vi "Basic Binding Test.vi"() -> (0 "error out":errorcluster)   [LabVIEW 2014, in "SQLite3LV Tests.lvlib"]
uses:
  SQLite3LV Tests.lvlib
  SQLite3LV/SQLite3 Class/struct_table_info.ctl
  SQLite3LV/Cursor Class/property binding/bind text.vi
  SQLite3LV/SQLite3 Class/sqlite3.lvclass
  SQLite3LV/Cursor Class/cursor.lvclass
  SQLite3LV/SQLite3LV.lvlib
panel:
  out "table info.":T1[](array[typedef])
  out "result":string[][](array[string])
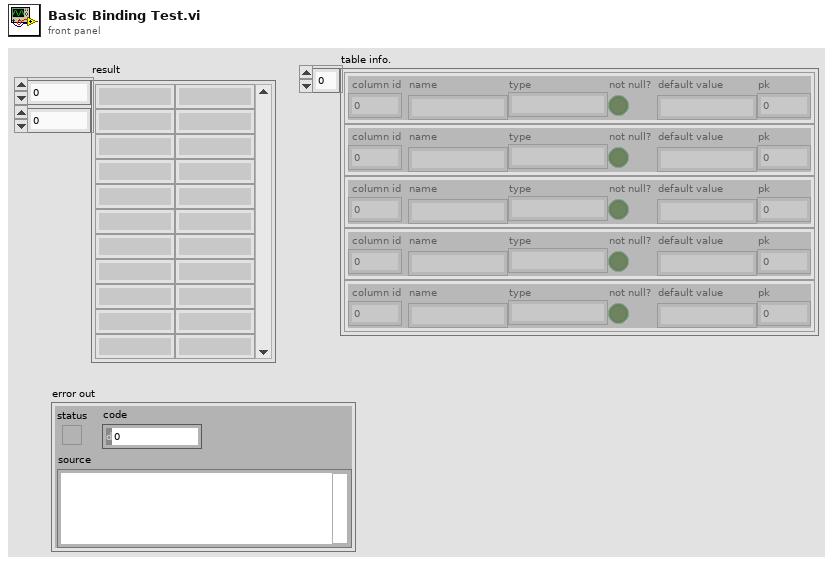
[diagram p1: front panel]
types:
  T1 = typedef "SQLite3LV.lvlib/struct_table_info.ctl" = cluster{" column id":i32, "name":string, "type":string, "not null?":bool, "default value":string, "pk":i32}
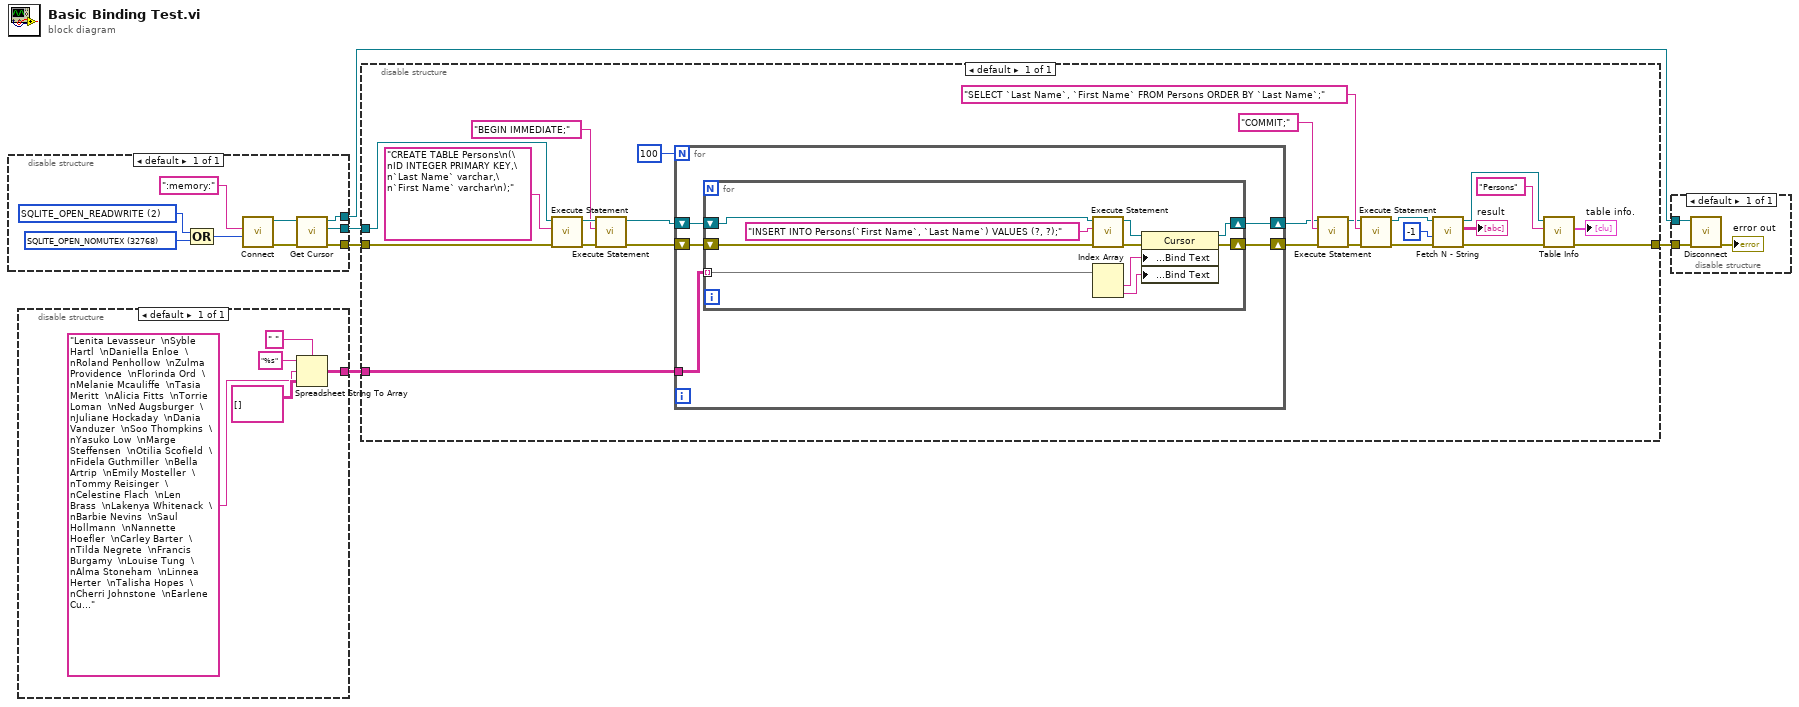
[diagram p0: block diagram]
diagram:
  n1 = disable-structure shown="default" {
    disable-tunnel: [w9] -> w5
    disable-tunnel: [w8] -> w4
    disable-tunnel: [w7] -> w3
    frame Enabled {
      w13 = u32 32768 items=["SQLITE_OPEN_READONLY"=1, "SQLITE_OPEN_READWRITE"=2, "SQLITE_OPEN_CREATE"=4, "SQLITE_OPEN_DELETEONCLOSE"=8, "SQLITE_OPEN_EXCLUSIVE"=16, "SQLITE_OPEN_AUTOPROXY"=32, "SQLITE_OPEN_URI"=64, "SQLITE_OPEN_MEMORY"=128, "SQLITE_OPEN_MAIN_DB"=256, "SQLITE_OPEN_TEMP_DB"=512, "SQLITE_OPEN_TRANSIENT_DB"=1024, "SQLITE_OPEN_MAIN_JOURNAL"=2048, "SQLITE_OPEN_TEMP_JOURNAL"=4096, "SQLITE_OPEN_SUBJOURNAL"=8192, "SQLITE_OPEN_MASTER_JOURNAL"=16384, "SQLITE_OPEN_NOMUTEX"=32768, "SQLITE_OPEN_FULLMUTEX"=65536, "SQLITE_OPEN_SHAREDCACHE"=131072, "SQLITE_OPEN_PRIVATECACHE"=262144, "SQLITE_OPEN_WAL"=524288] ("SQLITE3 Open Flag")
      w14 = u32 2 items=["SQLITE_OPEN_READONLY"=1, "SQLITE_OPEN_READWRITE"=2, "SQLITE_OPEN_CREATE"=4, "SQLITE_OPEN_DELETEONCLOSE"=8, "SQLITE_OPEN_EXCLUSIVE"=16, "SQLITE_OPEN_AUTOPROXY"=32, "SQLITE_OPEN_URI"=64, "SQLITE_OPEN_MEMORY"=128, "SQLITE_OPEN_MAIN_DB"=256, "SQLITE_OPEN_TEMP_DB"=512, "SQLITE_OPEN_TRANSIENT_DB"=1024, "SQLITE_OPEN_MAIN_JOURNAL"=2048, "SQLITE_OPEN_TEMP_JOURNAL"=4096, "SQLITE_OPEN_SUBJOURNAL"=8192, "SQLITE_OPEN_MASTER_JOURNAL"=16384, "SQLITE_OPEN_NOMUTEX"=32768, "SQLITE_OPEN_FULLMUTEX"=65536, "SQLITE_OPEN_SHAREDCACHE"=131072, "SQLITE_OPEN_PRIVATECACHE"=262144, "SQLITE_OPEN_WAL"=524288] ("SQLITE3 Open Flag")
      n2 = Compound Arithmetic op=OR(w14, w13) -> (w11:u32)
      n3 = call "Connect.vi"("SQLITE3 open flags"=w11, "path"=":memory:" ("path_utf8")) -> ("error out"=w6:errorcluster, "SQLite3LV Connection out"=w10:refnum<class "sqlite3.lvclass">)  [unwired: 8 in]
      n4 = call "Get Cursor.vi"("error in (no error)"=w6, "SQLite3LV Connection in"=w10) -> ("error out"=w7:errorcluster, "SQLite3LV Cursor"=w8:refnum<class "cursor.lvclass">, "SQLite3LV Connection out"=w9:refnum<class "sqlite3.lvclass">)  [unwired: 7 in]
    }
  }
  n5 = disable-structure shown="default" {
    disable-tunnel: [w15] -> w2
    frame Enabled {
      n6 = Spreadsheet String To Array(delimiter (Tab)=" ", format string="%s", spreadsheet string="Lenita Levasseur  \nSyble Hartl  \nDaniella Enloe  \nRoland Penhollow  \nZulma Providence  \nFlorinda Ord  \nMelanie Mcauliffe  \nTasia Meritt  \nAlicia Fitts  \nTorrie Loman  \nNed Augsburger  \nJuliane Hockaday  \nDania Vanduzer  \nSoo Thompkins  \nYasuko Low  \nMarge Steffensen  \nOtilia Scofield  \nFidela Guthmiller  \nBella Artrip  \nEmily Mosteller  \nTommy Reisinger  \nCelestine Flach  \nLen Brass  \nLakenya Whitenack  \nBarbie Nevins  \nSaul Hollmann  \nNannette Hoefler  \nCarley Barter  \nTilda Negrete  \nFrancis Burgamy  \nLouise Tung  \nAlma Stoneham  \nLinnea Herter  \nTalisha Hopes  \nCherri Johnstone  \nEarlene Culwell  \nFoster Binion  \nDolores Saxton  \nAshton Moody  \nShonta Fong  \nElicia Topping  \nZona Crigger  \nCaleb Poli  \nRosia Moton  \nShawanna Mcclure  \nRuthie Laguerre  \nStepanie Volz  \nGenesis Fullbright  \nFred Stam  \nIrene Santiago\nShenika Spieker  \nShanika Hogue  \nMarcus Ruppe  \nLaverne Gentry  \nWeston Ruiz  \nStefan Start  \nChelsie Wallen  \nCodi Lauderback  \nTerry Urman  \nEleanora Fujii  \nAugusta Lan  \nAlecia Mcgaugh  \nLynelle Capozzoli  \nDamien Mazzotta  \nCollin Janik  \nRene Binette  \nMelodee Vanderzee  \nShakia Brinkerhoff  \nSarita Wehner  \nElfriede Ashton  \nEllyn Taylor  \nAlia Kaplan  \nCandice Borgman  \nMari Pica  \nWillia Michaux  \nLucie Wilbourn  \nRoselee Villasenor  \nRebbeca Cadena  \nGolden Erazo  \nRoselle Saner  \nLetty Latimer  \nGeri Shives  \nOnie Ardon  \nRashida Sheroan  \nJenise Deford  \nSteven Doody  \nElnora Hose  \nNathanial Wardwell  \nSheila Hilyard  \nDarin Nieto  \nElida Jenney  \nLara Bona  \nWilburn Augusta  \nGrace Demarest  \nKeena Arzola  \nFidel Nusbaum  \nJanae Bissonnette  \nMartin Bibb  \nMerri Reading  \nIssac Degree", array type (2D Dbl)=string[][] []) -> (array=w15:string[][])
    }
  }
  n7 = disable-structure shown="default" {
    disable-tunnel: w4 -> [w40]
    disable-tunnel: w3 -> [w39]
    disable-tunnel: w2 -> [w38]
    disable-tunnel: [w33] -> w1
    frame Enabled {
      n8 = call "Execute Statement.vi"("error in (no error)"=w39, "SQL statement"="CREATE TABLE Persons\n(\nID INTEGER PRIMARY KEY,\n`Last Name` varchar,\n`First Name` varchar\n);" ("statement"), "SQLite3LV Cursor in"=w40) -> ("error out"=w29:errorcluster, "SQLite3LV Cursor out"=w30:refnum<class "cursor.lvclass">)  [unwired: 7 in]
      n9 = call "Execute Statement.vi"("error in (no error)"=w29, "SQL statement"="BEGIN IMMEDIATE;", "SQLite3LV Cursor in"=w30) -> ("error out"=w22:errorcluster, "SQLite3LV Cursor out"=w23:refnum<class "cursor.lvclass">)  [unwired: 7 in]
      n10 = for {
        N: 100 -> [_]
        tunnel: w38 -> [w49]
        shift-right: [w45] -> w21
        shift-left: w23 -> [w47]
        shift-right: [w48] -> w25
        shift-left: w22 -> [w46]
        n11 = for {
          shift-right: [w52] -> w45
          shift-left: w47 -> [w59]
          shift-right: [w51] -> w48
          shift-left: w46 -> [w57]
          tunnel: w49 -> [w54] mode=indexing
          n12 = call "Execute Statement.vi"("error in (no error)"=w57, "SQL statement"="INSERT INTO Persons(`First Name`, `Last Name`) VALUES (?, ?);" ("statement"), "SQLite3LV Cursor in"=w59) -> ("error out"=w56:errorcluster, "SQLite3LV Cursor out"=w55:refnum<class "cursor.lvclass">)  [unwired: 7 in]
          n13 = Index Array(array=w54) -> (element #1=w53:string, element #2=w50:string)  [unwired: 2 in]
          n14 = property class="Cursor"(reference=w55, error in=w56, "property binding:Bind Text"=w53, "property binding:Bind Text"=w50) -> (reference out=w52:refnum<class "cursor.lvclass">, error out=w51:errorcluster)
        }
      }
      n15 = call "Execute Statement.vi"("error in (no error)"=w25, "SQL statement"="COMMIT;", "SQLite3LV Cursor in"=w21) -> ("error out"=w26:errorcluster, "SQLite3LV Cursor out"=w27:refnum<class "cursor.lvclass">)  [unwired: 7 in]
      n16 = call "Execute Statement.vi"("error in (no error)"=w26, "SQL statement"="SELECT `Last Name`, `First Name` FROM Persons ORDER BY `Last Name`;" ("statement"), "SQLite3LV Cursor in"=w27) -> ("error out"=w41:errorcluster, "SQLite3LV Cursor out"=w42:refnum<class "cursor.lvclass">)  [unwired: 7 in]
      n17 = call "Fetch N - String.vi"("error in (no error)"=w41, "n rows (-1:all)"=-1, "SQLite3LV Cursor in"=w42) -> ("error out"=w35:errorcluster, "result"=→"result":string[][], "SQLite3LV Cursor out"=w34:refnum<class "cursor.lvclass">)  [unwired: 5 in, 1 out]
      n18 = call "Table Info.vi"("error in (no error)"=w35, "table"="Persons", "SQLite3LV Cursor in"=w34) -> ("error out"=w33:errorcluster, "table info."=→"table info.":T1[])  [unwired: 6 in, 1 out]
    }
  }
  n19 = disable-structure shown="default" {
    disable-tunnel: w5 -> [w61]
    disable-tunnel: w1 -> [w60]
    frame Enabled {
      n20 = call "Disconnect.vi"("error in (no error)"=w60, "SQLite3LV Connection in"=w61) -> ("error out"=→"error out":errorcluster)  [unwired: 9 in]
    }
  }
